vi "C3--End Sw.vi"(8 "Command Info In":T1, 10 "C3--End Sw":T4={"1a"=90.0, "1d"=45.31, "1s"=0.8, "2a"=180.0, "3t"=67.25, "4d"=0.65, "4s"=-90.0, "5a"=19.31, "6d"=0.5, "6s"=3.0}, 11 "Switch":string) -> (0 "Command Info Out":T1)   [LabVIEW 2017]
uses:
  Block Clusters/C3--End Sw.ctl
  <vilib>/Rock Robotics/WPI/Framework/Command Status Info.ctl
  <vilib>/Rock Robotics/WPI/Framework/Completion Status.ctl
  <vilib>/Rock Robotics/WPI/Framework/Completion Notifier.ctl
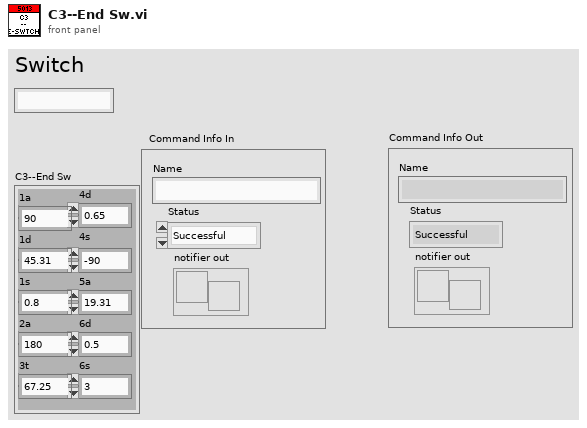
[diagram p1: front panel]
types:
  T1 = typedef "Command Status Info.ctl" = cluster{"Name":string, "Status":T2, "notifier out":T3}
  T2 = typedef "Completion Status.ctl" = enum16{"Successful", "Aborted", "Incomplete"}
  T3 = typedef "Completion Notifier.ctl" = refnum<notifier>
  T4 = typedef "C3--End Sw.ctl" = cluster{"1a":dbl, "1d":dbl, "1s":dbl, "2a":dbl, "3t":dbl, "4d":dbl, "4s":dbl, "5a":dbl, "6d":dbl, "6s":dbl}
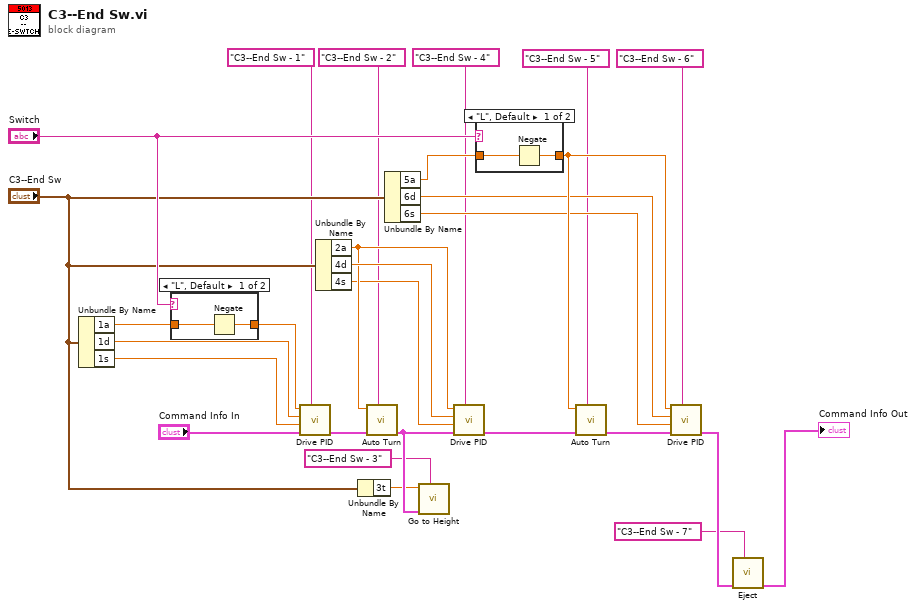
[diagram p0: block diagram]
diagram:
  n1 = Unbundle By Name("C3--End Sw") -> ("1a"=w26:dbl, "1d"=w25:dbl, "1s"=w23:dbl)
  n2 = case shown="\"L\", Default" "Switch" {
    tunnel: [w30 w31] -> w24
    tunnel: w26 -> [w29 w31]
    frame "L", Default {
      n3 = Negate(x=w29) -> (-x=w30:dbl)
    }
    frame "R" {
    }
  }
  n4 = call "Drive PID.vi"("Description"="C3--End Sw - 1", "Command Info In"="Command Info In", "Speed"=w23, "Distance"=w25, "Target Angle"=w24) -> ("Command Info Out"=w27:T1)  [unwired: 6 in]
  n5 = Unbundle By Name("C3--End Sw") -> ("2a"=w13:dbl, "4d"=w22:dbl, "4s"=w12:dbl)
  n6 = Unbundle By Name("C3--End Sw") -> ("3t"=w14:dbl)
  n7 = call "Auto Turn.vi"("Description"="C3--End Sw - 2", "Command Info In"=w27, "Target Angle"=w13) -> ("Command Info Out"=w21:T1)  [unwired: 8 in]
  n8 = Unbundle By Name("C3--End Sw") -> ("5a"=w10:dbl, "6d"=w9:dbl, "6s"=w8:dbl)
  n9 = call "Go to Height.vi"("Description"="C3--End Sw - 3", "Command Info In"=w21, "Target Height (in)"=w14) -> ()  [unwired: 8 in, 1 out]
  n10 = call "Drive PID.vi"("Description"="C3--End Sw - 4", "Command Info In"=w21, "Speed"=w12, "Distance"=w22, "Target Angle"=w13) -> ("Command Info Out"=w19:T1)  [unwired: 6 in]
  n11 = case shown="\"L\", Default" "Switch" {
    tunnel: [w33 w34] -> w20
    tunnel: w10 -> [w32 w34]
    frame "L", Default {
      n12 = Negate(x=w32) -> (-x=w33:dbl)
    }
    frame "R" {
    }
  }
  n13 = call "Auto Turn.vi"("Description"="C3--End Sw - 5", "Command Info In"=w19, "Target Angle"=w20) -> ("Command Info Out"=w18:T1)  [unwired: 8 in]
  n14 = call "Drive PID.vi"("Description"="C3--End Sw - 6", "Command Info In"=w18, "Speed"=w8, "Distance"=w9, "Target Angle"=w20) -> ("Command Info Out"=w17:T1)  [unwired: 6 in]
  n15 = call "Eject.vi"("Description"="C3--End Sw - 7", "Command Info In"=w17) -> ("Command Info Out"=→"Command Info Out":T1)  [unwired: 9 in]
